vi "Calculate R and G - Two Terminal.vi"(8 "Vsource":i32, 9 "Current":i32, 10 "AO Amp (V)":dbl[](array[numeric]) format="%.3p", 11 "Lockin []":dbl[](array[numeric])) -> (2 "G_2T (Siemens)":dbl, 3 "R_2T (Ohms)":dbl)   [LabVIEW 2016, in "Transport.lvclass"]
uses:
  Transport.lvclass
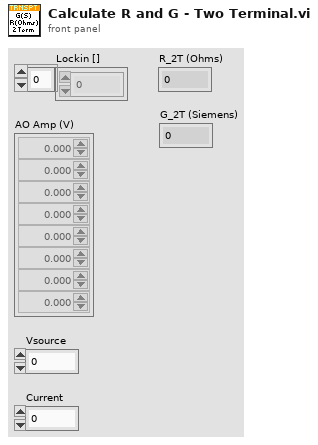
[diagram p1: front panel]
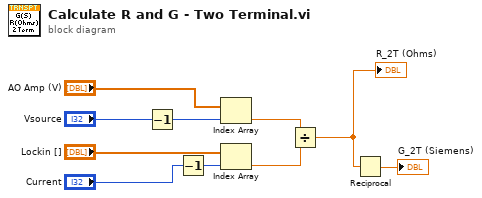
[diagram p0: block diagram]
diagram:
  n1 = Decrement(x="Vsource") -> (x-1=w5:i32)
  n2 = Decrement(x="Current") -> (x-1=w4:i32)
  n3 = Index Array(array="AO Amp (V)", index=w5) -> (element=w6:dbl)
  n4 = Index Array(array="Lockin []", index=w4) -> (element=w7:dbl)
  n5 = Divide(x=w6, y=w7) -> (x/y=w2:dbl)
  "R_2T (Ohms)" <- w2
  n6 = Reciprocal(x=w2) -> (1/x=→"G_2T (Siemens)":dbl)
